vi "Trig du Raman.vi"() -> ()   [LabVIEW 2010]
panel:
  in  "Boolean 2":bool=TRUE
  out "Numeric 2":i32
  out "Numeric":i32
  in  "Boolean":bool
  out "data":dynamicdata(graph)
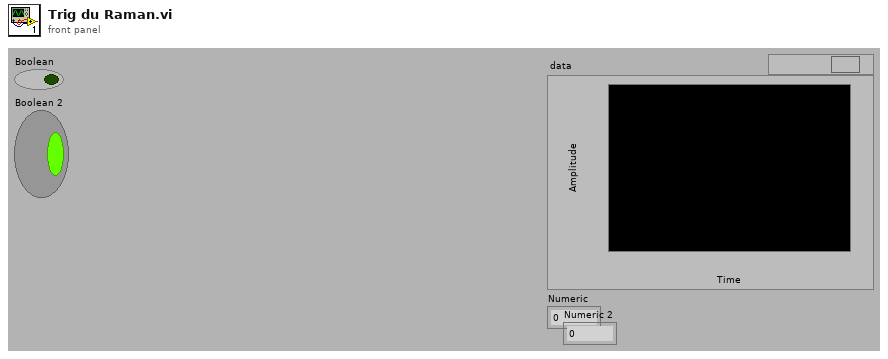
[diagram p1: front panel]
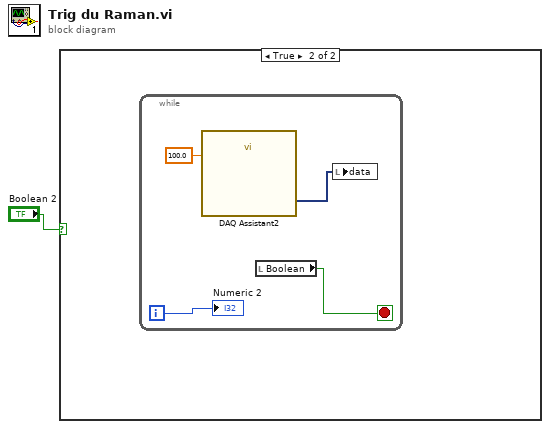
[diagram p0: block diagram]
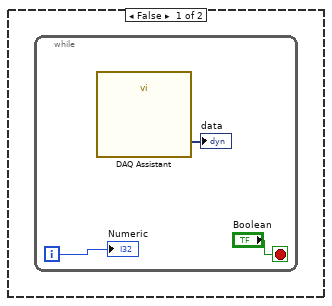
[diagram p2: hidden frame]
diagram:
  n1 = case shown="True" "Boolean 2" {
    frame False {
      n2 = while {
        i -> [w2]
        stop <- "Boolean" stop-if-true
        n3 = call "DAQ Assistant"() -> ("data"=→"data":dynamicdata)  [unwired: 16 in, 3 out]
        "Numeric" <- w2
      }
    }
    frame True {
      n4 = while {
        i -> [w8]
        stop <- w6 stop-if-true
        n5 = call "DAQ Assistant2"("timeout (s)"=100.0) -> ("data"=w7:dynamicdata)  [unwired: 16 in, 2 out]
        n6 = local read "Boolean"() -> (w6:bool)
        n7 = local write "data"(w7) -> ()
        "Numeric 2" <- w8
      }
    }
  }
